vi "check time.vi"(8 "error in (no error)":errorcluster, 11 "stopping criteria":T1={"function tolerance"=1e-06, "parameter tolerance"=1e-06, "max iterations"=0, "max function calls"=0, "gradient tolerance"=0.0, "max time (sec)"=1000.0, "initial tick count"=0}) -> (0 "error out":errorcluster)   [LabVIEW 2018, in "NI_Gmath.lvlib"]
uses:
  NI_Gmath.lvlib
  stopping criteria with time.ctl
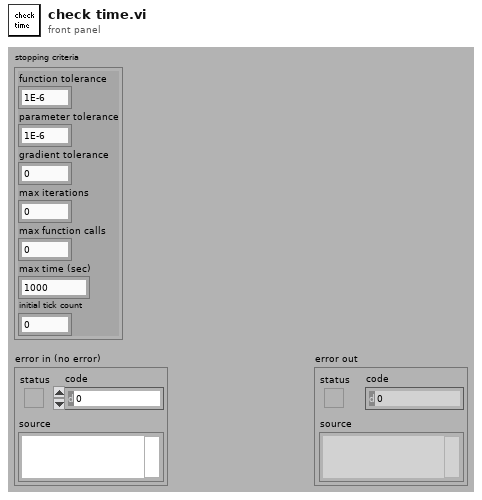
[diagram p1: front panel]
types:
  T1 = typedef "NI_Gmath.lvlib/stopping criteria with time.ctl" = cluster{"function tolerance":dbl, "parameter tolerance":dbl, "max iterations":i32, "max function calls":i32, "gradient tolerance":dbl, "max time (sec)":dbl, "initial tick count":u32}
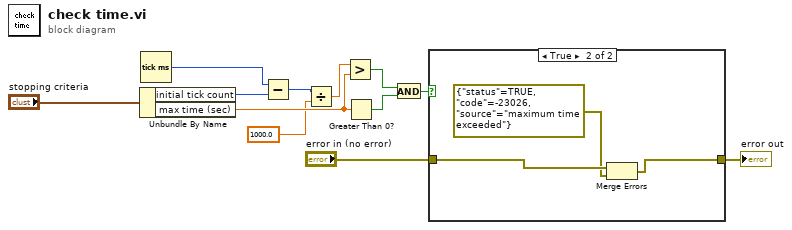
[diagram p0: block diagram]
diagram:
  n1 = Unbundle By Name("stopping criteria") -> ("initial tick count"=w5:u32, "max time (sec)"=w6:dbl)
  n2 = Tick Count (ms)() -> (millisecond timer value=w4:u32)
  n3 = Subtract(x=w4, y=w5) -> (x-y=w2:u32)
  n4 = Divide(x=w2, y=1000.0) -> (x/y=w1:dbl)
  n5 = Greater?(x=w1, y=w6) -> (0:w9:bool)
  n6 = Greater Than 0?(x=w6) -> (x > 0?=w10:bool)
  n7 = And(x=w9, y=w10) -> (x .and. y?=w8:bool)
  n8 = case shown="True" w8 {
    tunnel: "error in (no error)" -> [w13 w16]
    tunnel: [w13 w15] -> w11
    frame False {
    }
    frame True {
      n9 = Merge Errors(w16, errorcluster {"status"=TRUE, "code"=-23026, "source"="maximum time exceeded"} ("error out")) -> (w15:errorcluster)
    }
  }
  "error out" <- w11
